vi "flattenToString.vi"(8 "error in (no error)":errorcluster, 10 "Record":refnum<class "Record.lvclass">, 11 "Serializer in":refnum<class "Serializer.lvclass">) -> (0 "error out":errorcluster, 2 "Flattened String":string, 3 "Serializer out":refnum<class "Serializer.lvclass">)   [LabVIEW 2017, in "Error Log.lvlib" / "Serializer.lvclass"]
uses:
  Serializer.lvclass
  Record/Record.lvclass
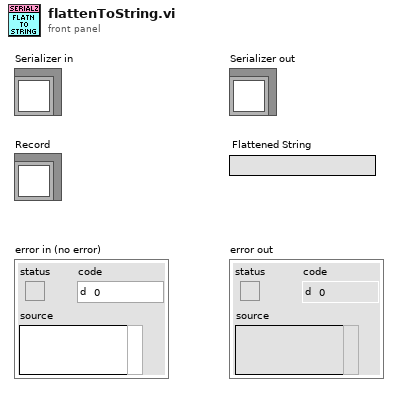
[diagram p1: front panel]
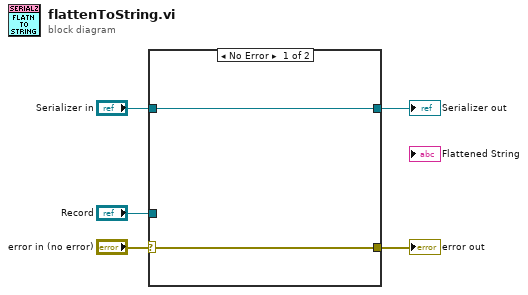
[diagram p0: block diagram]
diagram:
  n1 = case shown="No Error" "error in (no error)" {
    selector: "error in (no error)" -> [w6 w9]
    tunnel: [w6 w9] -> w4
    tunnel: [w7 w8] -> w2
    tunnel: "Serializer in" -> [w7 w8]
    tunnel: "Record" -> [_ _]
    frame No Error {
    }
    frame Error {
    }
  }
  "error out" <- w4
  "Serializer out" <- w2
